vi "BuildingQueryDeleteRecipeInFunctionToParameters.vi"(9 "dataReadingToDelete":T1, 10 "dataReadingOut":string[][](array[string]), 11 "columns":string[](array[string])) -> (3 "queryToDelete":string)   [LabVIEW 2014]
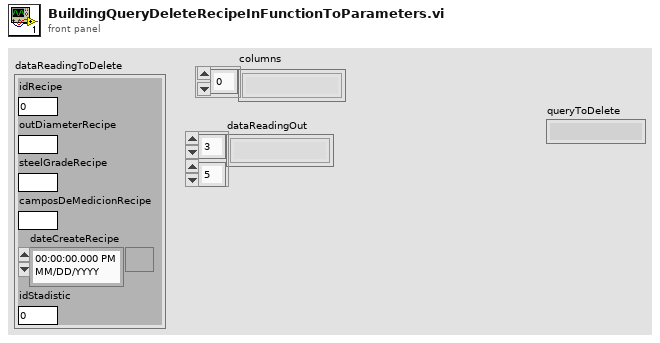
[diagram p1: front panel]
types:
  T1 = cluster{"idRecipe":dbl, "outDiameterRecipe":string, "steelGradeRecipe":string, "camposDeMedicionRecipe":string, "dateCreateRecipe":timestamp, "idStadistic":dbl}
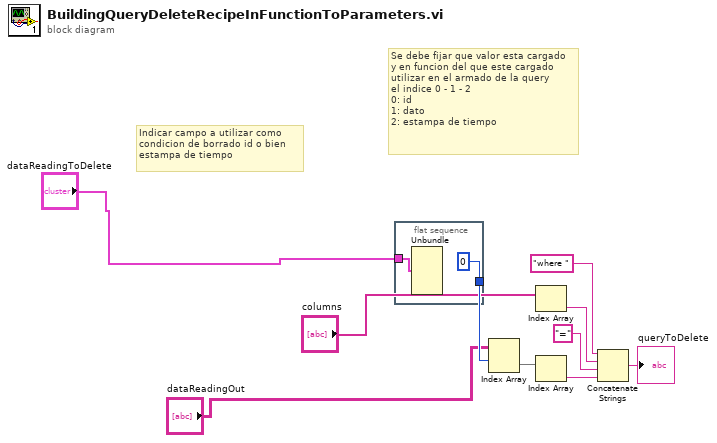
[diagram p0: block diagram]
diagram:
  # "Se debe fijar que valor esta cargado\ny en funcion del que este cargado \nutilizar en el armado de la query \nel indice 0 - 1 - 2 \n0: id\n1: dato\n2: estampa de tiempo"
  # "Indicar campo a utilizar como \ncondicion de borrado id o bien\nestampa de tiempo"
  n1 = flat-sequence {
    tunnel: "dataReadingToDelete" -> [w12]
    tunnel: [0 ("index")] -> w5
    frame #0 {
      n2 = Unbundle(w12) -> ()  [unwired: 6 out]
    }
  }
  n3 = Index Array(array="dataReadingOut", index (row)=w5) -> (element=w6:string[])  [unwired: 1 in]
  n4 = Index Array(array="columns") -> (element=w9:string)  [unwired: 1 in]
  n5 = Index Array(array=w6) -> (element=w10:string)  [unwired: 1 in]
  n6 = Concatenate Strings("where " ("condition"), w9, "=" ("string"), w10) -> (→"queryToDelete":string)
